vi "readTCPDataIn v1.vi"(0 "TCP Network Connection in":refnum<k5>, 5 "Size of data":string, 11 "error in (no error)":errorcluster) -> (4 "TCP Network Connection out":refnum<k5>, 6 "Operation":string, 8 "Operation+Data":string, 10 "Data":string, 15 "error out":errorcluster)   [LabVIEW 2015]
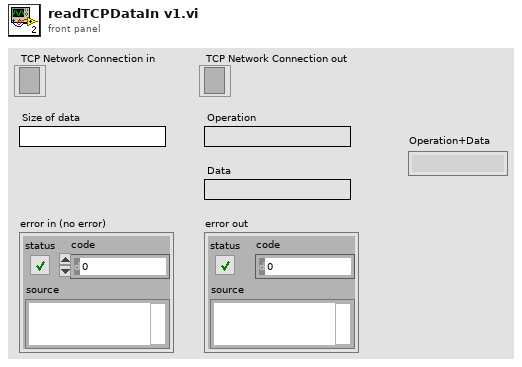
[diagram p1: front panel]
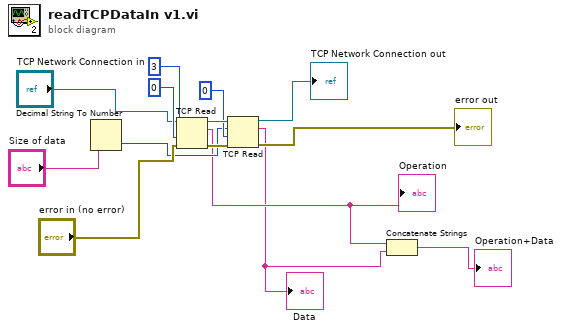
[diagram p0: block diagram]
diagram:
  n1 = Decimal String To Number(string="Size of data") -> (number=w8:i32)  [unwired: 2 in, 1 out]
  n2 = TCP Read(connection ID="TCP Network Connection in", bytes to read=3, error in (no error)="error in (no error)", 9:0 ("timeout ms (25000)")) -> (connection ID out=w10:refnum<k5>, data out=w3:string, error out=w12:errorcluster)  [unwired: 1 in]
  "Operation" <- w3
  n3 = TCP Read(connection ID=w10, bytes to read=w8, error in (no error)=w12, 9:0 ("timeout ms (25000)")) -> (connection ID out=→"TCP Network Connection out":refnum<k5>, data out=w2:string, error out=→"error out":errorcluster)  [unwired: 1 in]
  "Data" <- w2
  n4 = Concatenate Strings(w3, w2) -> (→"Operation+Data":string)
